vi "EXIF UI.vi"() -> ()   [LabVIEW 2023, in "EXIF Modifier.lvlib"]
uses:
  EXIF Modifier.lvlib
  Controls/exif_producer cluster.ctl
  Controls/exif_consumer cluster.ctl
  Controls/exif_info cluster.ctl
  <vilib>/Utility/miscctls.llb/LVRowAndColumnTypeDef.ctl
panel:
  out "Status":string
  in  "Set DateTimeOrginal":timestamp format="%<%Y-%m-%d %H:%M:%S>T"
  out "Selected Photo DateTimeOrginal":timestamp format="%<%Y-%m-%d %H:%M:%S>T"
  in  "Apply":bool
  in  "Preview":bool
  in  "Reload":bool
  in  "Folder Path":path
  in  "Listbox":i32(listbox)
  in  "Producer Cluster In":T1
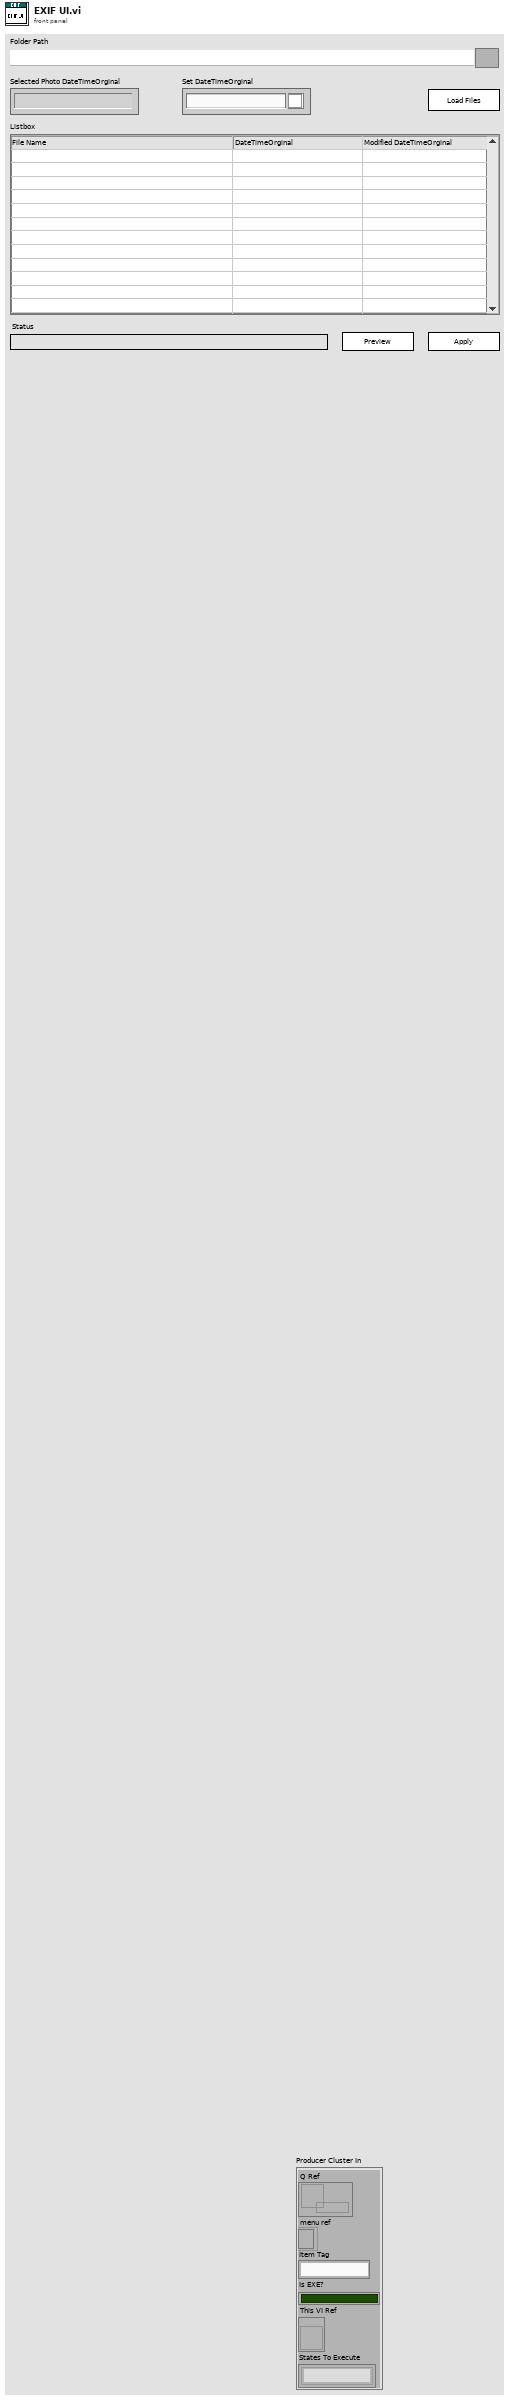
[diagram p1: front panel]
types:
  T1 = typedef "EXIF Modifier.lvlib/exif_producer cluster.ctl" = cluster{"Q Ref":refnum<queue>, "menu ref":refnum<k9>, "Item Tag":string, "Is EXE?":bool, "This VI Ref":refnum<vi>, "States To Execute":string[]}
  T2 = typedef "EXIF Modifier.lvlib/exif_consumer cluster.ctl" = cluster{"Running VI":refnum<vi>, "Test VI":refnum<vi>, "Q Ref":refnum<queue>, "UE":refnum<event-registration>, "Data":variant, "Timeout":i32, "ListBox[]":string[][], "Source Path":path, "Delta Time":dbl, "ExifInfo[]":T3[], "ListIndex":i32, "counter":i32, "Format":enum16{"Files Only", "Files Date", "All"}, "total":i32, "Operation":enum16{"Read Info", "Write Info"}, "Status":string}
  T3 = typedef "EXIF Modifier.lvlib/exif_info cluster.ctl" = cluster{"DateTimeOrginal":timestamp, "FilePath":path, "New DateTime":timestamp, "FileName":string}
  T4 = typedef "LVRowAndColumnTypeDef.ctl" = cluster{"Row":i32, "Column":i32}
  T5 = enum32{"invalid app kind", "Development System", "Run Time System", "Student Edition", "Embedded LabVIEW", "Evaluation", "Custom"}
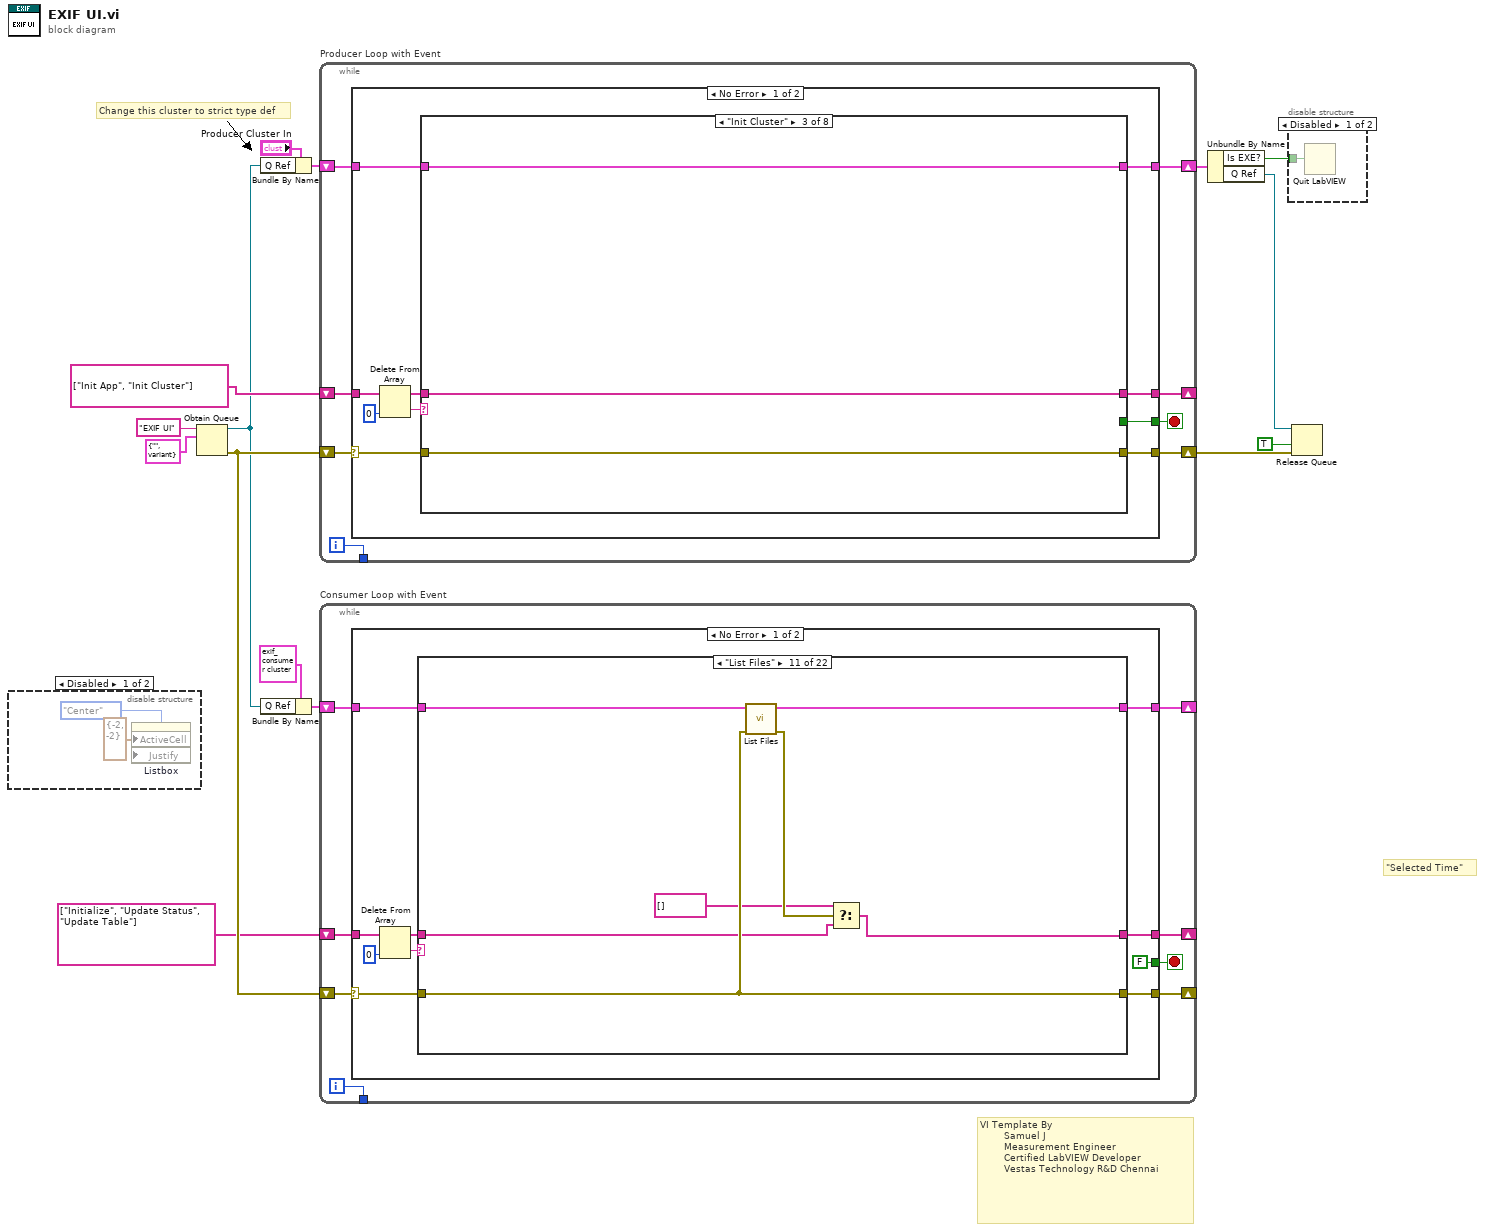
[diagram p0: block diagram]
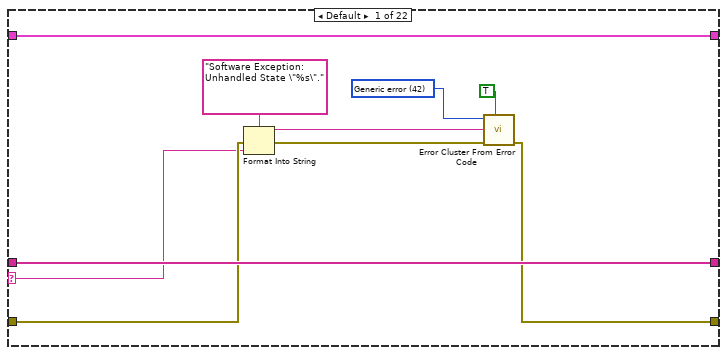
[diagram p4: hidden frame]
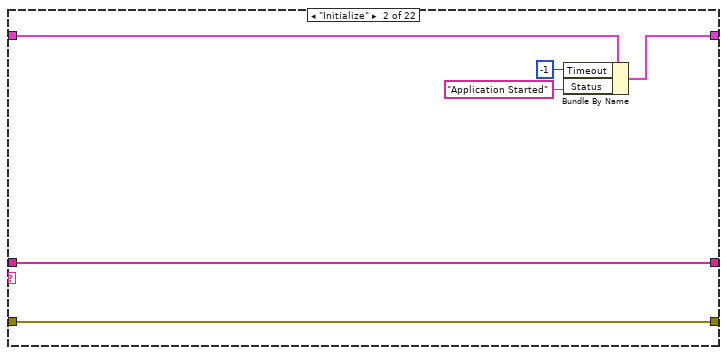
[diagram p5: hidden frame]
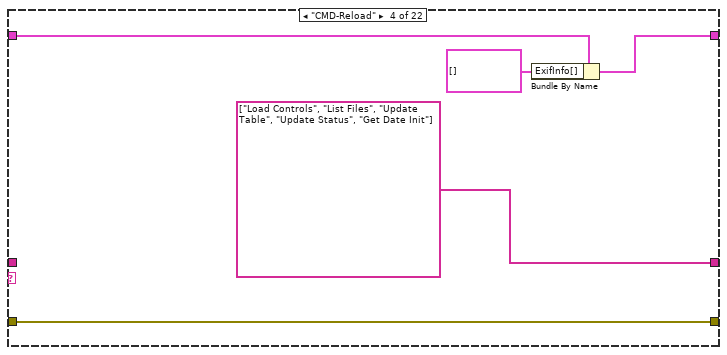
[diagram p7: hidden frame]
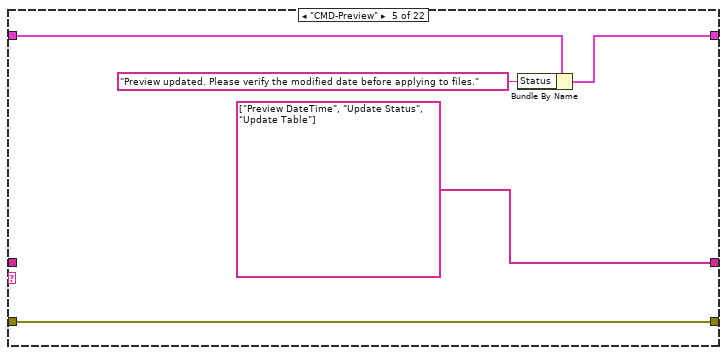
[diagram p8: hidden frame]
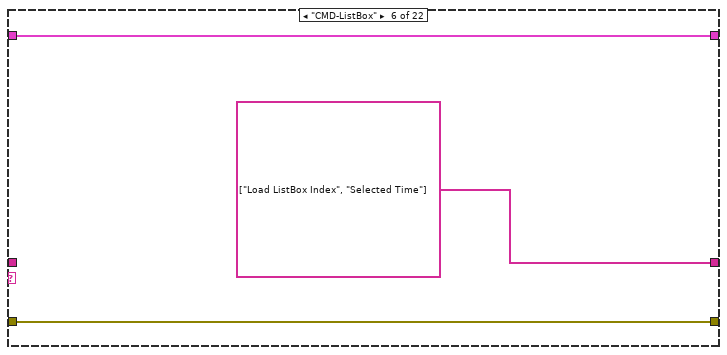
[diagram p9: hidden frame]
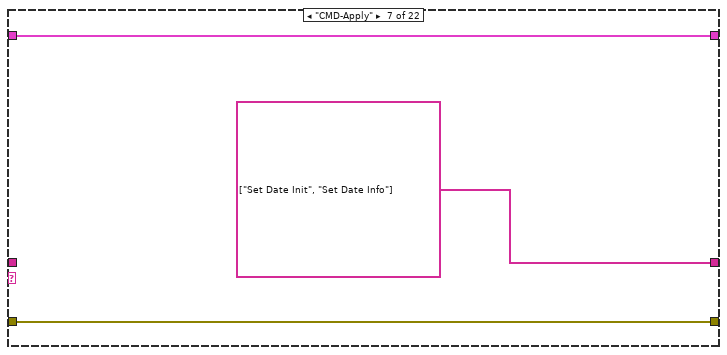
[diagram p10: hidden frame]
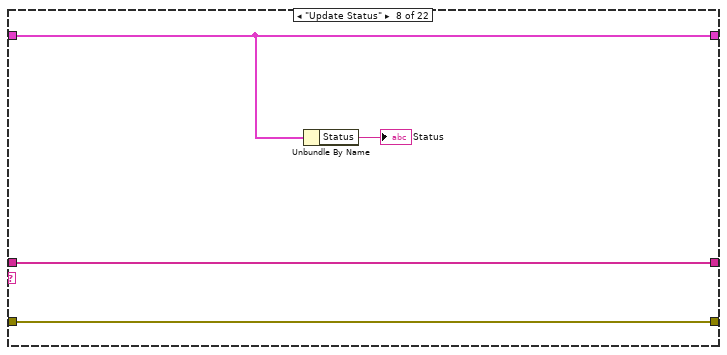
[diagram p11: hidden frame]
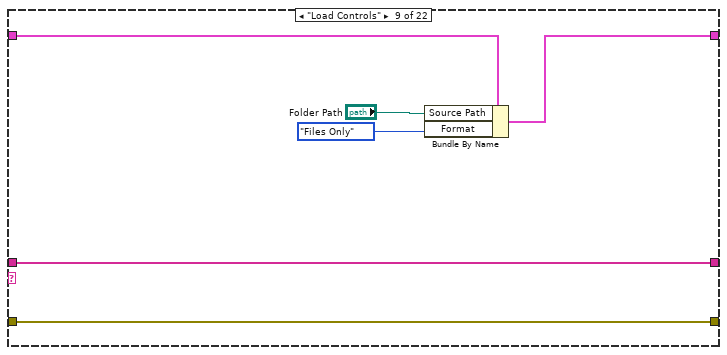
[diagram p12: hidden frame]
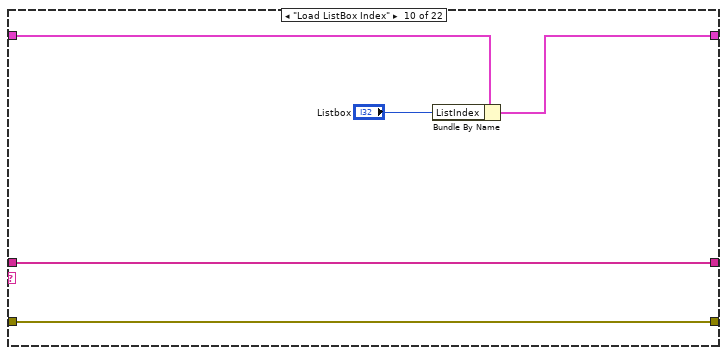
[diagram p13: hidden frame]
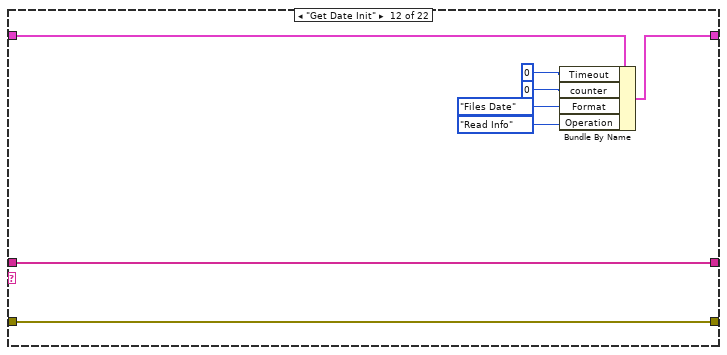
[diagram p14: hidden frame]
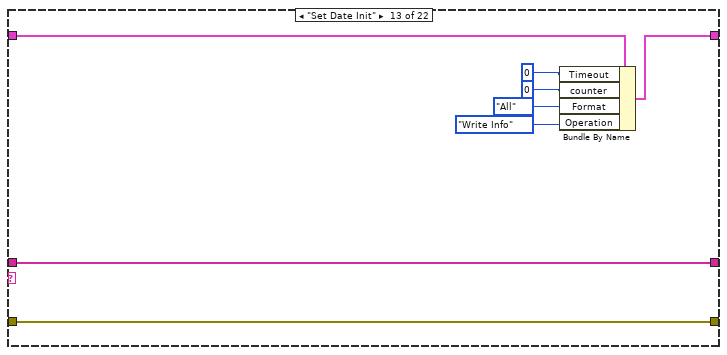
[diagram p15: hidden frame]
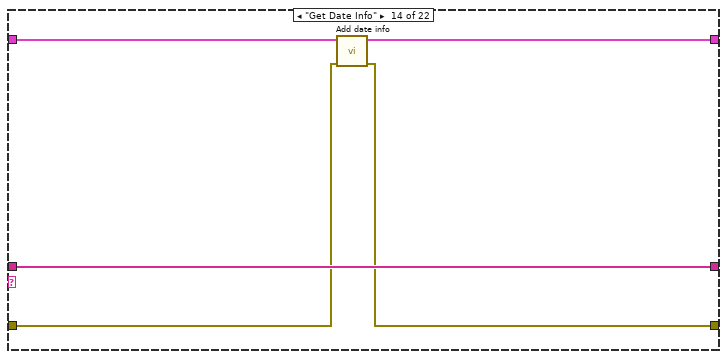
[diagram p16: hidden frame]
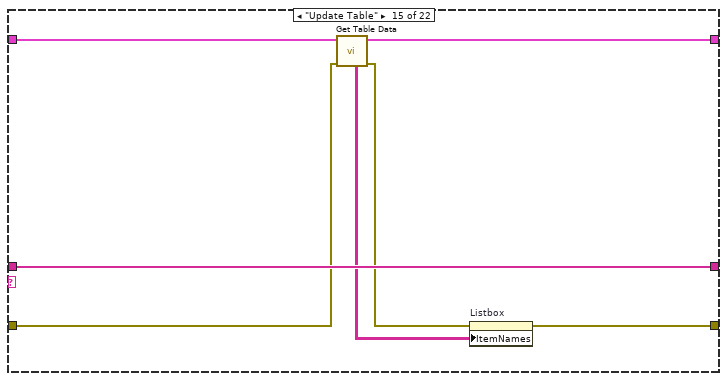
[diagram p17: hidden frame]
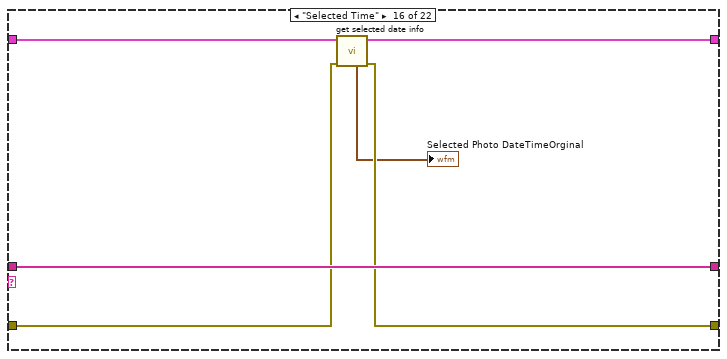
[diagram p18: hidden frame]
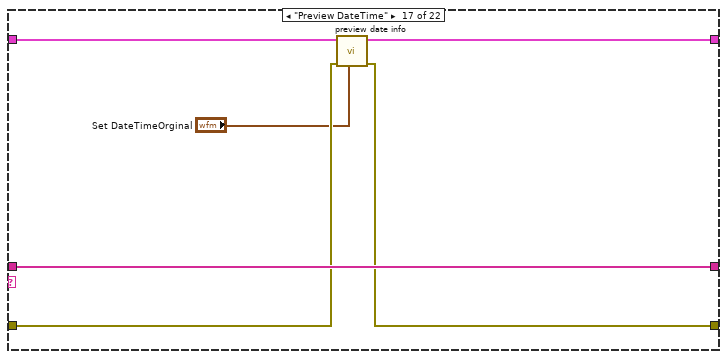
[diagram p19: hidden frame]
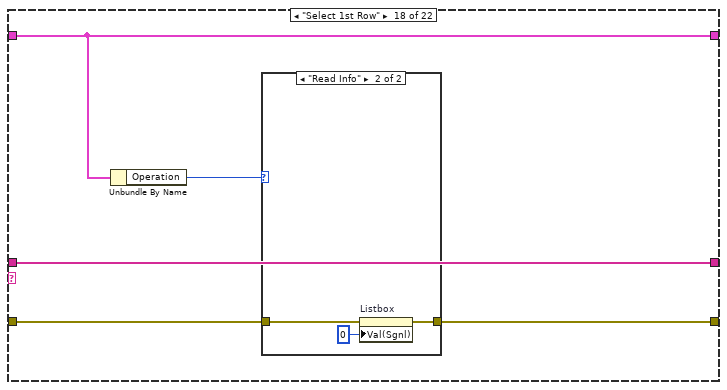
[diagram p20: hidden frame]
diagram:
  # "\"Selected Time\""
  # "Change this cluster to strict type def"
  # "VI Template By\n        Samuel J\n        Measurement Engineer\n        Certified LabVIEW Developer\n        Vestas Technology R&D Chennai"
  n1 = disable-structure shown="Disabled" {
    frame Disabled {
      n2 = property on="Listbox" class="MCListbox (strict)"("ActiveCell"=T4 {"Row"=-2, "Column"=-2} ("Active Cell:Active Cell"), "Justify"=enum16{"Left", "Center", "Right"}."Center" ("Active Cell:Cell Justification")) -> ()  [unwired: 2 in, 2 out]
    }
    frame Enabled {
    }
  }
  n3 = Obtain Queue(name (unnamed)="EXIF UI", element data type=cluster{"Command":string, "Data":variant} {"Command"="", "Data"=variant} ("Data Cluster")) -> (queue out=w11:refnum<queue>, error out=w12:errorcluster)  [unwired: 3 in, 1 out]
  n4 = Bundle By Name(cluster="Producer Cluster In", "Q Ref"=w11) -> (w4:T1)
  n5 = Bundle By Name(cluster=T2 {"Running VI"=refnum, "Test VI"=refnum, "Q Ref"=refnum, "UE"=refnum, "Data"=variant, "Timeout"=-1, "ListBox[]"=[], "Source Path"=path "", "Delta Time"=0.0, "ExifInfo[]"=[], "ListIndex"=0, "counter"=0, "Format"=enum."Files Only", "total"=0, "Operation"=enum."Read Info", "Status"=""} ("Consumer Cluster in"), "Q Ref"=w11) -> (w13:T2)
  n6 = while "Producer Loop with Event" {
    shift-right: [w24] -> w2
    shift-left: w12 -> [w25]
    shift-right: [w21] -> _
    shift-left: string[] ["Init App", "Init Cluster"] ("appended array") -> [w22]
    shift-right: [w19] -> w5
    shift-left: w4 -> [w20]
    tunnel: [w18] -> _
    i -> [w18]
    stop <- w23 stop-if-true
    n7 = case shown="No Error" w25 {
      selector: w25 -> [w35 w131]
      tunnel: [w34 w135] -> w24
      tunnel: [w33 FALSE] -> w23
      tunnel: w22 -> [w32 _]
      tunnel: [w28 string[] []] -> w21
      tunnel: w20 -> [w27 w130]
      tunnel: [w26 w130] -> w19
      frame No Error {
        n8 = Delete From Array(array=w32, index=0) -> (deleted portion=w30:string, array with subset deleted=w29:string[])  [unwired: 1 in]
        n9 = case shown="\"Init Cluster\"" w30 {
          selector: w30 -> [w38 _ _ _ _ _ _ _]
          tunnel: w35 -> [w40 w52 w61 w66 w82 w116 w121 w126]
          tunnel: [w39 w47 w61 w64 w81 w116 w121 w126] -> w34
          tunnel: [FALSE FALSE _ FALSE ("T button?") FALSE ("T button?") _ FALSE TRUE ("T button?")] -> w33
          tunnel: w29 -> [w46 w57 w60 w69 w80 w115 w122 w128]
          tunnel: [w46 w57 w60 w69 w79 w115 w122 w128] -> w28
          tunnel: w27 -> [w37 w58 w59 w67 w77 w114 w118 w125]
          tunnel: [w37 w55 w59 w67 w78 w114 w118 w125] -> w26
          frame Default {
            w42 = 42 items=["No error", "Argument error", "Memory is full", "Out of zone", "End of file", "File already open", "Generic file I/O error", "File not found", "File permission error", "Disk is full", "Duplicate path", "Too many files open", "System feature not enabled", "Resource file not found", "Cannot add resource", "Resource not found", "Image not found", "Image memory error", "Pen does not exist", "Config type invalid", "Config token not found", "Config parse error", "Config memory error", "Bad external code format", "Bad external code offset", "External code not present", "Null window", "Destroy window error", "Null menu", "Print aborted", "Bad print record", "Print driver error", "Windows error during printing", "Memory error during printing", "Print dialog error", "Generic print error", "Invalid device refnum", "Device not found", "Device parameter error", "Device unit error", "Cannot open device", "Device call aborted", "Generic error", "Cancelled by user", "Object ID too low", "Object ID too high", "Object not in heap", "Unknown heap", "Unknown object (invalid DefProc)", "Unknown object (DefProc not in table)", "Message out of range", "Invalid (null) method", "Unknown message", "Manager call not supported", "Bad address", "Network operation in progress", "Network operation timed out", "Connection is busy", "Network attribute not supported", "Network error", "Address in use", "System out of memory", "Connection aborted", "Connection refused", "Not connected", "Already connected", "Connection closed", "Initialization error (interapplication manager)", "Bad occurrence", "Wait on unbound occurrence handler", "Occurrence queue overflow", "Datalog type conflict", "Unused", "Unrecognized type (interapplication manager)", "Memory corrupt", "Failed to make temporary DLL", "Old CIN version", "Drag socket not found", "Failed to load drop-object", "Failed to register OLE object", "Failed to release OLE object", "Format specifier type mismatch", "Unknown format specifier", "Too few format specifiers", "Too many format specifiers", "Scan failed", "Newer CIN version", "Error converting to variant", "Runtime menu error", "Password tampered", "Variant attribute not found", "Incompatible variant data type", "Event data is not available", "Event Store is not present", "Occurrence is not found", "Event Queue is not created", "Event info is not available", "Refnum passed is NULL", "Error retrieving Class GUID", "Error retrieving CoClass GUID", "Error retrieving TypeLib GUID.", "Bad built application magic bytes.", "Specific driver is different from the specific driver associated with the Logical Name.", "There is no session opened to the class driver.", "Max Error", "MAX - Error with config objects", "MAX - Error loading configuration", "MAX - Group not supported"]
            n10 = Format Into String(format string="Software Exception: Unhandled State \"%s\"." ("message"), error in=w40, w38) -> (resulting string=w43:string, error out=w44:errorcluster)  [unwired: 1 in]
            n11 = call <vilib>:"Error Cluster From Error Code.vi"("show call chain? (False)"=TRUE, "error in (no error)"=w44, "error message (\"\")"=w43, "error code (0)"=w42) -> ("error out"=w39:errorcluster)  [unwired: 5 out]
          }
          frame "Init App" {
            n12 = property class="App"(error in=w52) -> (error out=w48:errorcluster, "App.Kind"=w50:T5)  [unwired: 1 in, 1 out]
            n13 = control-ref of="This VI"() -> (w53:refnum<vi>)
            n14 = Equal?(x=w50, y=T5."Run Time System" ("Application:Kind")) -> (x = y?=w49:bool)
            n15 = Current VI's Menubar() -> (w54:refnum<k9>)
            n16 = Bundle By Name(cluster=w58, "menu ref"=w54, "This VI Ref"=w53, "Is EXE?"=w49) -> (w55:T1)
            n17 = call <userlib>:"Set Pane Orgin 00.vi"("error in"=w48) -> ("error out"=w47:errorcluster)  [unwired: 10 in]
          }
          frame "Init Cluster" {
          }
          frame "Enqueue" {
            n18 = Unbundle By Name(w67) -> ("Q Ref"=w65:refnum<queue>, "States To Execute"=w63:string[])
            n19 = for {
              tunnel: w65 -> [w74]
              shift-right: [w73] -> w64
              shift-left: w66 -> [w75]
              tunnel: w63 -> [w72] mode=indexing
              tunnel: variant ("Data") -> [w71]
              n20 = Bundle("element"=w72, "Data"=w71) -> (w70:cluster{"element":string, "Data":variant})  [unwired: 1 in]
              n21 = Enqueue Element(queue=w74, element=w70, error in (no error)=w75) -> (error out=w73:errorcluster)  [unwired: 1 in, 2 out]
            }
          }
          frame "", "Events" {
            n22 = event shown="[3] \"Listbox\": Value Change" {
              selector: _ -> [_ _ _ _ _ _ _]
              dyn-events: _ -> [_ _ _ _ _ _ _]
              timeout: _ -> [_ _ _ _ _ _ _]
              tunnel: w82 -> [w86 w89 w94 w99 w104 w109 w113]
              tunnel: [w86 w89 w94 w99 w104 w109 w113] -> w81
              tunnel: w80 -> [_ _ _ _ _ _ _]
              tunnel: [string[] ["EXIT"] string[] [] string[] ["Enqueue"] ("appended array") string[] ["Enqueue"] ("appended array") string[] ["Enqueue"] ("appended array") string[] ["Enqueue"] ("appended array") w110] -> w79
              tunnel: [w85 w88 w91 w96 w101 w106 w112] -> w78
              tunnel: w77 -> [w85 w88 w92 w97 w102 w107 w112]
              event Panel Close? {
                n23 = event-data() -> ()  [unwired: 2 out]
                n24 = event-data("Discard?"=TRUE) -> ()  [unwired: 1 in, 1 out]
              }
              event Timeout {
                n25 = event-data() -> ()  [unwired: 2 out]
              }
              event "Reload": Value Change {
                n26 = event-data() -> ()  [unwired: 2 out]
                n27 = Bundle By Name(cluster=w92, "States To Execute"=string[] ["CMD-Reload"] ("appended array")) -> (w91:T1)
              }
              event "Listbox": Value Change {
                n28 = event-data() -> ()  [unwired: 2 out]
                n29 = Bundle By Name(cluster=w97, "States To Execute"=string[] ["CMD-ListBox"] ("appended array")) -> (w96:T1)
              }
              event "Apply": Value Change {
                n30 = event-data() -> ()  [unwired: 7 out]
                n31 = Bundle By Name(cluster=w102, "States To Execute"=string[] ["CMD-Apply"] ("appended array")) -> (w101:T1)
              }
              event "Preview": Value Change {
                n32 = event-data() -> ()  [unwired: 2 out]
                n33 = Bundle By Name(cluster=w107, "States To Execute"=string[] ["CMD-Preview"] ("appended array")) -> (w106:T1)
              }
              event Menu Selection (User) {
                n34 = event-data() -> ("ItemTag"=w111:string)  [unwired: 1 out]
                n35 = Build Array(w111) -> (w110:string[])
              }
            }
          }
          frame "--------- EVENTS ---------" {
            # "Don't delete this case\nTo add a event case duplicate this case and add case selector"
          }
          frame "CONTEXT_HELP" {
            # "Toggle Show/Hide Context Help Window"
            n36 = fn#1354() -> (1:w119:bool)  [unwired: 1 out]
            n37 = Not(x=w119) -> (.not. x?=w120:bool)
            n38 = Control Help Window(1:w120) -> ()  [unwired: 1 out]
          }
          frame "EXIT" {
            n39 = Unbundle By Name(w125) -> ("This VI Ref"=w123:refnum<vi>, "Is EXE?"=w124:bool)
            n40 = case shown="True" w124 {
              tunnel: w123 -> [_ w129]
              frame False {
              }
              frame True {
                n41 = invoke class="VI" method="FP.Close"(reference=w129) -> ()  [unwired: 2 in, 3 out]
              }
            }
          }
        }
      }
      frame Error {
        n42 = Unbundle By Name(w131) -> ("code"=w132:i32)
        n43 = case shown="42" w132 {
          tunnel: [w137 w139] -> w136
          tunnel: w131 -> [w137 w138]
          frame Default {
          }
          frame 42 {
            # "State Error"
            n44 = call <vilib>:"Simple Error Handler.vi"("error in (no error)"=w138) -> ("error out"=w139:errorcluster)  [unwired: 1 in, 7 out]
          }
        }
        n45 = call <vilib>:"Clear Errors.vi"("error in (no error)"=w136) -> ("error out"=w135:errorcluster)  [unwired: 1 in, 5 out]
      }
    }
  }
  n46 = while "Consumer Loop with Event" {
    shift-right: [w146] -> _
    shift-left: w12 -> [w147]
    shift-right: [w143] -> _
    shift-left: string[] ["Initialize", "Update Status", "Update Table"] ("appended array") -> [w144]
    shift-right: [w141] -> _
    shift-left: w13 -> [w142]
    tunnel: [w140] -> _
    i -> [w140]
    stop <- w145 stop-if-true
    n47 = case shown="No Error" w147 {
      selector: w147 -> [w157 w311]
      tunnel: [w156 w314] -> w146
      tunnel: [FALSE w308] -> w145
      tunnel: w144 -> [w155 _]
      tunnel: [w151 string[] []] -> w143
      tunnel: w142 -> [w150 w312]
      tunnel: [w149 w312] -> w141
      frame No Error {
        n48 = Delete From Array(array=w155, index=0) -> (deleted portion=w153:string, array with subset deleted=w152:string[])  [unwired: 1 in]
        n49 = case shown="\"List Files\"" w153 {
          selector: w153 -> [w159 _ _ _ _ _ _ _ _ _ _ _ _ _ _ _ _ _ _ _ _ _]
          tunnel: w157 -> [w161 w172 w176 w181 w186 w189 w192 w196 w202 w207 w211 w222 w230 w232 w240 w245 w251 w258 w265 w271 w291 w306]
          tunnel: [w160 w172 w176 w181 w186 w189 w192 w196 w202 w207 w211 w222 w230 w231 w237 w244 w250 w257 w264 w270 w291 w305] -> w156
          tunnel: w152 -> [w167 w173 w175 _ _ _ _ w195 w201 w206 w210 w221 w229 w235 w242 w248 w254 w259 w268 w282 _ _]
          tunnel: [w167 w173 w175 string[] ["Load Controls", "List Files", "Update Table", "Update Status", "Get Date Init"] ("f") string[] ["Preview DateTime", "Update Status", "Update Table"] ("f") string[] ["Load ListBox Index", "Selected Time"] ("f") string[] ["Set Date Init", "Set Date Info"] ("f") w195 w201 w206 w209 w221 w229 w235 w242 w248 w254 w259 w268 w282 w283 w297] -> w151
          tunnel: w150 -> [w158 w171 w174 w179 w184 w188 w191 w193 w200 w205 w214 w220 w228 w234 w241 w247 w253 w256 w267 w278 w287 w303]
          tunnel: [w158 w170 w174 w178 w183 w188 w191 w193 w199 w204 w213 w219 w227 w233 w236 w246 w252 w256 w266 w279 w287 w302] -> w149
          frame Default {
            w163 = 42 items=["No error", "Argument error", "Memory is full", "Out of zone", "End of file", "File already open", "Generic file I/O error", "File not found", "File permission error", "Disk is full", "Duplicate path", "Too many files open", "System feature not enabled", "Resource file not found", "Cannot add resource", "Resource not found", "Image not found", "Image memory error", "Pen does not exist", "Config type invalid", "Config token not found", "Config parse error", "Config memory error", "Bad external code format", "Bad external code offset", "External code not present", "Null window", "Destroy window error", "Null menu", "Print aborted", "Bad print record", "Print driver error", "Windows error during printing", "Memory error during printing", "Print dialog error", "Generic print error", "Invalid device refnum", "Device not found", "Device parameter error", "Device unit error", "Cannot open device", "Device call aborted", "Generic error", "Cancelled by user", "Object ID too low", "Object ID too high", "Object not in heap", "Unknown heap", "Unknown object (invalid DefProc)", "Unknown object (DefProc not in table)", "Message out of range", "Invalid (null) method", "Unknown message", "Manager call not supported", "Bad address", "Network operation in progress", "Network operation timed out", "Connection is busy", "Network attribute not supported", "Network error", "Address in use", "System out of memory", "Connection aborted", "Connection refused", "Not connected", "Already connected", "Connection closed", "Initialization error (interapplication manager)", "Bad occurrence", "Wait on unbound occurrence handler", "Occurrence queue overflow", "Datalog type conflict", "Unused", "Unrecognized type (interapplication manager)", "Memory corrupt", "Failed to make temporary DLL", "Old CIN version", "Drag socket not found", "Failed to load drop-object", "Failed to register OLE object", "Failed to release OLE object", "Format specifier type mismatch", "Unknown format specifier", "Too few format specifiers", "Too many format specifiers", "Scan failed", "Newer CIN version", "Error converting to variant", "Runtime menu error", "Password tampered", "Variant attribute not found", "Incompatible variant data type", "Event data is not available", "Event Store is not present", "Occurrence is not found", "Event Queue is not created", "Event info is not available", "Refnum passed is NULL", "Error retrieving Class GUID", "Error retrieving CoClass GUID", "Error retrieving TypeLib GUID.", "Bad built application magic bytes.", "Specific driver is different from the specific driver associated with the Logical Name.", "There is no session opened to the class driver.", "Max Error", "MAX - Error with config objects", "MAX - Error loading configuration", "MAX - Group not supported"]
            n50 = Format Into String(format string="Software Exception: Unhandled State \"%s\"." ("message"), error in=w161, w159) -> (resulting string=w164:string, error out=w165:errorcluster)  [unwired: 1 in]
            n51 = call <vilib>:"Error Cluster From Error Code.vi"("show call chain? (False)"=TRUE, "error in (no error)"=w165, "error message (\"\")"=w164, "error code (0)"=w163) -> ("error out"=w160:errorcluster)  [unwired: 5 out]
          }
          frame "Initialize" {
            n52 = Bundle By Name(cluster=w171, "Timeout"=-1, "Status"="Application Started") -> (w170:T2)
          }
          frame "---------- COMMAND  ----------" {
          }
          frame "CMD-Reload" {
            n53 = Bundle By Name(cluster=w179, "ExifInfo[]"=T3[] []) -> (w178:T2)
          }
          frame "CMD-Preview" {
            n54 = Bundle By Name(cluster=w184, "Status"="Preview updated. Please verify the modified date before applying to files.") -> (w183:T2)
          }
          frame "CMD-ListBox" {
          }
          frame "CMD-Apply" {
          }
          frame "Update Status" {
            n55 = Unbundle By Name(w193) -> ("Status"=→"Status":string)
          }
          frame "Load Controls" {
            n56 = Bundle By Name(cluster=w200, "Source Path"="Folder Path", "Format"=enum16{"Files Only", "Files Date", "All"}."Files Only") -> (w199:T2)
          }
          frame "Load ListBox Index" {
            n57 = Bundle By Name(cluster=w205, "ListIndex"="Listbox") -> (w204:T2)
          }
          frame "List Files" {
            n58 = call "List Files.vi"("error in"=w211, "Cluster in"=w214) -> ("error out"=w212:errorcluster, "Cluster out"=w213:T2)  [unwired: 8 in]
            n59 = Select(t=string[] [], s=w212, f=w210) -> (s? t:f=w209:string[])
          }
          frame "Get Date Init" {
            n60 = Bundle By Name(cluster=w220, "Timeout"=0 ("timeout"), "counter"=0, "Format"=enum16{"Files Only", "Files Date", "All"}."Files Date", "Operation"=enum16{"Read Info", "Write Info"}."Read Info") -> (w219:T2)
          }
          frame "Set Date Init" {
            n61 = Bundle By Name(cluster=w228, "Timeout"=0 ("timeout"), "counter"=0, "Format"=enum16{"Files Only", "Files Date", "All"}."All", "Operation"=enum16{"Read Info", "Write Info"}."Write Info") -> (w227:T2)
          }
          frame "Get Date Info" {
            n62 = call "Add date info.vi"("error in"=w232, "Cluster in"=w234) -> ("error out"=w231:errorcluster, "Cluster out"=w233:T2)  [unwired: 8 in]
          }
          frame "Update Table" {
            n63 = call "Get Table Data.vi"("error in"=w240, "Cluster in"=w241) -> ("error out"=w238:errorcluster, "Cluster out"=w236:T2, "Table[]"=w239:string[][])  [unwired: 7 in]
            n64 = property on="Listbox" class="MCListbox (strict)"(error in=w238, "ItemNames"=w239) -> (error out=w237:errorcluster)  [unwired: 1 in, 1 out]
          }
          frame "Selected Time" {
            n65 = call "get selected date info.vi"("error in"=w245, "Cluster in"=w247) -> ("error out"=w244:errorcluster, "Cluster out"=w246:T2, "DateTimeOrginal"=→"Selected Photo DateTimeOrginal":timestamp)  [unwired: 7 in]
          }
          frame "Preview DateTime" {
            n66 = call "preview date info.vi"("DateTimeOrginal"="Set DateTimeOrginal", "error in"=w251, "Cluster in"=w253) -> ("error out"=w250:errorcluster, "Cluster out"=w252:T2)  [unwired: 7 in]
          }
          frame "Select 1st Row" {
            n67 = Unbundle By Name(w256) -> ("Operation"=w255:enum16{"Read Info", "Write Info"})
            n68 = case shown="\"Read Info\"" w255 {
              tunnel: w258 -> [w260 w263]
              tunnel: [w260 w262] -> w257
              frame "Write Info", Default {
              }
              frame "Read Info" {
                n69 = property on="Listbox" class="MCListbox (strict)"(error in=w263, "Val(Sgnl)"=0 ("Value (Signaling)")) -> (error out=w262:errorcluster)  [unwired: 1 in, 1 out]
              }
            }
          }
          frame "Set Date Info" {
            n70 = call "apply new date info.vi"("error in"=w265, "Cluster in"=w267) -> ("error out"=w264:errorcluster, "Cluster out"=w266:T2)  [unwired: 8 in]
          }
          frame "Stop Loop" {
            n71 = Unbundle By Name(w278) -> ("Operation"=w273:enum16{"Read Info", "Write Info"}, "total"=w277:i32)
            n72 = Equal To 0?(x=w273) -> (x = 0?=w276:bool)
            n73 = Select(t="Finished reading date info from all %d files." ("resulting string"), s=w276, f="Finished writing date info to all %d files." ("resulting string")) -> (s? t:f=w275:string)
            n74 = Format Into String(format string=w275, error in=w271, w277) -> (resulting string=w269:string, error out=w270:errorcluster)  [unwired: 1 in]
            n75 = Bundle By Name(cluster=w278, "Timeout"=-1 ("timeout"), "counter"=0, "Status"=w269) -> (w279:T2)
          }
          frame "Timeout" {
            n76 = Unbundle By Name(w287) -> ("counter"=w290:i32, "total"=w289:i32, "Operation"=w288:enum16{"Read Info", "Write Info"})
            n77 = Greater?(x=w290, y=w289) -> (0:w286:bool)
            n78 = case shown="\"Write Info\"" w288 {
              tunnel: [string[] ["Set Date Info", "Update Table", "Update Status"] ("appended array") string[] ["Get Date Info", "Update Table", "Update Status"] ("appended array")] -> w284
              frame "Write Info" {
              }
              frame "Read Info" {
              }
            }
            n79 = Select(t=string[] ["Stop Loop", "Update Status", "Select 1st Row"] ("appended array"), s=w286, f=w284) -> (s? t:f=w283:string[])
          }
          frame "", "Events" {
            # "Waiting for the command to execute\nIf timeout occurs timeout case executes"
            n80 = Unbundle By Name(w303) -> ("Q Ref"=w307:refnum<queue>, "Timeout"=w301:i32)
            n81 = Dequeue Element(queue=w307, timeout in ms (-1)=w301, error in (no error)=w306) -> (element=w304:cluster{"Command":string, "Data":variant}, timed out?=w298:bool, error out=w305:errorcluster)  [unwired: 1 out]
            n82 = Unbundle By Name(w304) -> ("Data"=w299:variant, "Command"=w300:string)
            n83 = Not(x=w298) -> (.not. x?=w295:bool)
            n84 = Bundle By Name(cluster=w303, "Data"=w299) -> (w302:T2)
            n85 = Build Array(w300) -> (w296:string[])
            n86 = Select(t=w296, s=w295, f=string[] ["Timeout"]) -> (s? t:f=w297:string[])
          }
        }
      }
      frame Error {
        n87 = Unbundle By Name(w311) -> ("code"=w309:i32)
        n88 = case shown="1, 1122" w309 {
          tunnel: w311 -> [w316 w318]
          tunnel: [w316 w317] -> w310
          tunnel: [TRUE FALSE] -> w308
          frame 1, 1122 {
          }
          frame Default {
            n89 = call <vilib>:"Simple Error Handler.vi"("error in (no error)"=w318) -> ("error out"=w317:errorcluster)  [unwired: 4 in, 4 out]
          }
        }
        n90 = call <vilib>:"Clear Errors.vi"("error in (no error)"=w310) -> ("error out"=w314:errorcluster)  [unwired: 1 in, 5 out]
      }
    }
  }
  n91 = Unbundle By Name(w5) -> ("Is EXE?"=w14:bool, "Q Ref"=w6:refnum<queue>)
  n92 = disable-structure shown="Disabled" {
    disable-tunnel: w14 -> [w320 _]
    frame Disabled {
      n93 = Quit LabVIEW(quit? (T)=w320) -> ()
    }
    frame Enabled {
    }
  }
  n94 = Release Queue(queue=w6, force destroy? (F)=TRUE, error in (no error)=w2) -> ()  [unwired: 3 out]
